vi "Control_Sensing_Sep.vi"() -> ()   [LabVIEW 2019]
uses:
  Control 1.ctl
  <vilib>/myRIO/Instrument Drivers/Onboard IO/I2C/typedefs/I2C User Configuration.ctl
  <vilib>/myRIO/Instrument Drivers/Onboard IO/I2C/typedefs/I2C Transfer Rate.ctl
  <vilib>/myRIO/Instrument Drivers/Onboard IO/I2C/typedefs/I2C Reference.ctl
  <vilib>/myRIO/Common/Instrument Driver Framework/Utilities/typedefs/myRIO Generic Hardware Reference.ctl
  <vilib>/myRIO/Common/Instrument Driver Framework/Utilities/typedefs/Hardware Version Enum.ctl
  <vilib>/myRIO/Common/Instrument Driver Framework/Utilities/typedefs/myRIO v1.0 Reference.ctl
  <vilib>/myRIO/Common/Instrument Driver Framework/Utilities/typedefs/Generic FPGA Reference.ctl
  <vilib>/myRIO/Common/Instrument Driver Framework/myRIO v1.0/I2C/typedefs/I2C Channels Enum.ctl
  <vilib>/myRIO/Instrument Drivers/Onboard IO/I2C/typedefs/I2C Configuration.ctl
  <vilib>/userDefined/High Color/nirio_resource_hc.ctl
  <vilib>/myRIO/Instrument Drivers/Onboard IO/AI/typedefs/AI Reference.ctl
  <vilib>/myRIO/Common/Instrument Driver Framework/myRIO v1.0/AI/typedefs/AI Channels List.ctl
  <vilib>/myRIO/Common/Instrument Driver Framework/myRIO v1.0/AI/typedefs/AI Channels Enum.ctl
  <vilib>/myRIO/Common/Instrument Driver Framework/Utilities/typedefs/Analog Scaling Constants List.ctl
  <vilib>/myRIO/Common/Instrument Driver Framework/Utilities/typedefs/Analog Scaling Constants.ctl
  <vilib>/myRIO/Instrument Drivers/Onboard IO/PWM/typedefs/PWM Reference.ctl
  <vilib>/myRIO/Common/Instrument Driver Framework/myRIO v1.0/PWM/typedefs/PWM Channels Enum.ctl
  <vilib>/myRIO/Instrument Drivers/Onboard IO/PWM/typedefs/PWM Configuration.ctl
  <vilib>/myRIO/Instrument Drivers/Onboard IO/DIO/typedefs/DIO Reference.ctl
  <vilib>/myRIO/Common/Instrument Driver Framework/myRIO v1.0/DIO/typedefs/DIO Channels List.ctl
  <vilib>/myRIO/Common/Instrument Driver Framework/myRIO v1.0/DIO/typedefs/DIO Channels Enum.ctl
  <vilib>/myRIO/Common/Instrument Driver Framework/Utilities/vis/Is FPGA Ref Available.vi
  <vilib>/myRIO/Common/Instrument Driver Framework/myRIO v1.0/I2C/vis/myRIO v1.1 Open I2C.vi
  <vilib>/myRIO/Instrument Drivers/Onboard IO/I2C/vis/Configure.vi
  <vilib>/myRIO/Instrument Drivers/Onboard IO/I2C/vis/Write.vi
  <vilib>/myRIO/Common/Instrument Driver Framework/myRIO v1.0/AI/vis/myRIO v1.1 Open AI.vi
  <vilib>/myRIO/Instrument Drivers/Onboard IO/AI/vis/Read.vi
  <vilib>/myRIO/Common/Instrument Driver Framework/myRIO v1.0/DIO/vis/myRIO v1.1 Open DIO.vi
  <vilib>/myRIO/Instrument Drivers/Onboard IO/DIO/vis/Write.vi
  <vilib>/myRIO/Common/Instrument Driver Framework/myRIO v1.0/PWM/vis/myRIO v1.1 Open PWM.vi
  <vilib>/myRIO/Instrument Drivers/Onboard IO/PWM/vis/Set Duty Cycle and Frequency.vi
  <vilib>/myRIO/Instrument Drivers/Onboard IO/I2C/vis/Write Read.vi
  <vilib>/myRIO/Common/Instrument Driver Framework/myRIO v1.0/UART/vis/myRIO v1.0 Close UART.vi
  <vilib>/myRIO/Common/Instrument Driver Framework/Utilities/vis/Validate Channels.vi
  <vilib>/myRIO/Common/Instrument Driver Framework/myRIO v1.0/I2C/vis/myRIO v1.0 Reserve I2C.vi
  <vilib>/myRIO/Common/Instrument Driver Framework/myRIO v1.0/AI/vis/myRIO v1.0 Reserve AI.vi
  <vilib>/myRIO/Common/Instrument Driver Framework/myRIO v1.0/DIO/vis/myRIO v1.0 Reserve DIO.vi
  <vilib>/myRIO/Common/Instrument Driver Framework/myRIO v1.0/PWM/vis/myRIO v1.0 Reserve PWM.vi
  <vilib>/myRIO/Common/Instrument Driver Framework/myRIO v1.0/I2C/vis/myRIO v1.0 Build MUX Configuration I2C.vi
  <vilib>/myRIO/Common/Instrument Driver Framework/myRIO v1.0/Resource Manager/vis/myRIO v1.0 Reserve Channel List.vi
  <vilib>/myRIO/Common/Instrument Driver Framework/myRIO v1.0/AI/vis/myRIO v1.0 Build MUX Configuration AI.vi
  <vilib>/myRIO/Common/Instrument Driver Framework/myRIO v1.0/DIO/vis/myRIO v1.0 Build MUX Configuration DIO.vi
  <vilib>/myRIO/Common/Instrument Driver Framework/myRIO v1.0/PWM/vis/myRIO v1.0 Build MUX Configuration PWM.vi
  <vilib>/myRIO/Common/Instrument Driver Framework/myRIO v1.0/Resource Manager/vis/myRIO v1.0 Create Configuration List.vi
  <vilib>/myRIO/Common/Instrument Driver Framework/myRIO v1.0/Resource Manager/vis/myRIO v1.0 Reserve Channel.vi
  <vilib>/myRIO/Common/Instrument Driver Framework/myRIO v1.0/Resource Manager/vis/myRIO v1.0 Unreserve Channel.vi
  <vilib>/myRIO/Common/Instrument Driver Framework/myRIO v1.0/Resource Manager/vis/myRIO v1.0 Build Mutex Name.vi
  <vilib>/imath/engines/lvmath2/RunTimeEngine/NodeEndStatement/NIMS_NodeEndStatement_Output.vi
  <instcachedir>/0/NIMS_NodeEndStatement_Output_53EC0D466D134D7ABD903AC30B43404B.lvgen/NIMS_NodeEndStatement_Output_53EC0D466D134D7ABD903AC30B43404B_000.vi
  <instcachedir>/0/NIMS_NodeEndStatement_Output_53EC0D466D134D7ABD903AC30B43404B.lvgen/NIMS_NodeEndStatement_Output_53EC0D466D134D7ABD903AC30B43404B_005.vi
  <vilib>/imath/engines/lvmath2/RunTimeEngine/ErrorHandling/NIMS_Finalize Error.vi
  <vilib>/imath/engines/lvmath2/RunTimeEngine/BuiltInFunctions/length/NIMS_length(GV).vi
  <instcachedir>/0/NIMS_length(GV)_08A3D13377FD4E4B96F5795FBF3698FA.lvgen/NIMS_length(GV)_08A3D13377FD4E4B96F5795FBF3698FA_000.vi
  <vilib>/imath/engines/lvmath2/RunTimeEngine/BuiltInFunctions/ones/NIMS_V=ones(I32,I32).vi
  <vilib>/imathl/engines/lvmath/Functions/Error Handling/Create Error.vi
  <vilib>/imath/engines/lvmath2/RunTimeEngine/RangeToken/NIMS_Range.vi
  <instcachedir>/0/NIMS_Range_FADF6ADDA3E145BB934C8BD4C7DAAB97.lvgen/NIMS_Range_FADF6ADDA3E145BB934C8BD4C7DAAB97_000.vi
  <vilib>/imath/engines/lvmath2/RunTimeEngine/Managers/WorkSpace/UID Generator.vi
  <vilib>/imath/engines/lvmath2/RunTimeEngine/RunTimeType/NIMS_RunTimeType_From StrictType (excl LVString).vi
  <instcachedir>/0/NIMS_RunTimeType_From StrictType (excl LVString)_D8AFBA86A94845AAA577C895450664BD.lvgen/NIMS_RunTimeType_From StrictType (excl LVString)_D8AFBA86A94845AAA577C895450664BD_000.vi
  <vilib>/imath/engines/lvmath2/RunTimeEngine/LocalVariableDefStatement/MC_LocalVariableDefStatement_Display.vi
  <vilib>/imath/engines/lvmath2/RunTimeEngine/BuiltInFunctions/diag/NIMS_diag.vi
  <instcachedir>/0/NIMS_diag_DCAB8C8FDAF64F9E84492BB524435AA9.lvgen/NIMS_diag_DCAB8C8FDAF64F9E84492BB524435AA9_003.vi
  <vilib>/imath/engines/lvmath2/RunTimeEngine/BuiltInFunctions/mirrorh/NIMS_mirrorh(GM).vi
  <instcachedir>/0/NIMS_mirrorh(GM)_A650AD0D730A4A8EBE251B4C5C7CA115.lvgen/NIMS_mirrorh(GM)_A650AD0D730A4A8EBE251B4C5C7CA115_004.vi
  <vilib>/imath/engines/lvmath2/RunTimeEngine/RowToken/NIMS_RowToken_M_M.vi
  <instcachedir>/0/NIMS_RowToken_M_M_21FE36D058524603B8B587AC30FD72C2.lvgen/NIMS_RowToken_M_M_21FE36D058524603B8B587AC30FD72C2_005.vi
  <vilib>/imath/engines/lvmath2/RunTimeEngine/ErrorHandling/NIMS_Create Error From Enums.vi
  <vilib>/imath/engines/lvmath2/RunTimeEngine/Managers/SymbolTable/Clear UID.vi
  <instcachedir>/0/NIMS_NodeEndStatement_Output_53EC0D466D134D7ABD903AC30B43404B.lvgen/NIMS_NodeEndStatement_Output_53EC0D466D134D7ABD903AC30B43404B_002.vi
  <instcachedir>/0/NIMS_NodeEndStatement_Output_53EC0D466D134D7ABD903AC30B43404B.lvgen/NIMS_NodeEndStatement_Output_53EC0D466D134D7ABD903AC30B43404B_010.vi
  <vilib>/Utility/VariantDataType/GetNumericInfo.vi
  <vilib>/Utility/error.llb/Error Cluster From Error Code.vi
  <vilib>/myRIO/Common/Instrument Driver Framework/myRIO v1.0/myRIO v1.1 Open.vi
  <vilib>/myRIO/Common/Instrument Driver Framework/Utilities/vis/IO Manager.vi
  <vilib>/myRIO/Common/Instrument Driver Framework/Utilities/vis/Configuration Manager.vi
  <vilib>/myRIO/Common/Instrument Driver Framework/myRIO v1.0/Resource Manager/vis/myRIO v1.0 Configure IO.vi
  <vilib>/myRIO/Common/Instrument Driver Framework/myRIO v1.0/myRIO v1.0 Close.vi
  <vilib>/myRIO/Common/Instrument Driver Framework/myRIO v1.0/I2C/vis/myRIO v1.0 Configure I2C.vi
  <vilib>/myRIO/Common/Instrument Driver Framework/myRIO v1.0/I2C/vis/myRIO v1.0 Write I2C.vi
  <vilib>/myRIO/Common/Instrument Driver Framework/myRIO v1.0/AI/vis/myRIO v1.0 Get Scaling Constants AI.vi
  <vilib>/myRIO/Common/Instrument Driver Framework/myRIO v1.0/AI/vis/myRIO v1.0 Read AI.vi
  <vilib>/myRIO/Common/Instrument Driver Framework/myRIO v1.0/PWM/vis/myRIO v1.0 Write PWM.vi
  <vilib>/myRIO/Common/Instrument Driver Framework/myRIO v1.0/DIO/vis/myRIO v1.0 Write DIO.vi
  <vilib>/myRIO/Common/Instrument Driver Framework/myRIO v1.0/I2C/vis/myRIO v1.0 Read I2C.vi
  OneDrive/Documents/LabVIEW Data/MathScriptVIs/MCStatic_41946317732_39d282e6f644b4de5e03d5ec5e14f762.vi
  <instcachedir>/0/MCStatic_41946317732_39d282e6f644b4de5e03d5ec5e14f762_F82D6288F92F4DD7BE24A1113A5A915E.lvgen/MCStatic_41946317732_39d282e6f644b4de5e03d5ec5e14f762_F82D6288F92F4DD7BE24A1113A5A915E_000.vi
  <vilib>/imath/engines/lvmath2/RunTimeEngine/ArithmeticOperatorToken/NIMS_ArithmeticOperator_multmx.vi
  <instcachedir>/0/NIMS_ArithmeticOperator_multmx_77F1D2D6F4D94BA7A97C4E7185C02392.lvgen/NIMS_ArithmeticOperator_multmx_77F1D2D6F4D94BA7A97C4E7185C02392_003.vi
  <instcachedir>/0/NIMS_diag_DCAB8C8FDAF64F9E84492BB524435AA9.lvgen/NIMS_diag_DCAB8C8FDAF64F9E84492BB524435AA9_002.vi
  <vilib>/imath/engines/lvmath2/RunTimeEngine/BuiltInFunctions/max/1 input/NIMS_max(CM).vi
  <instcachedir>/0/NIMS_max(CM)_ECFF9CEF2CF74B92B05BC258ECD38873.lvgen/NIMS_max(CM)_ECFF9CEF2CF74B92B05BC258ECD38873_000.vi
  <vilib>/imath/engines/lvmath/Functions/Error Handling/MergeErrorsWrapper.vi
  <vilib>/imath/engines/lvmath2/RunTimeEngine/CommandStatement/MC_CommandStatement_break.vi
  OneDrive/Documents/LabVIEW Data/MathScriptVIs/MCStatic_41946317732_3e71c9587ee176df8890ce07400746a8.vi
  <instcachedir>/0/MCStatic_41946317732_3e71c9587ee176df8890ce07400746a8_07A171384687481495CD1245C64FEFFE.lvgen/MCStatic_41946317732_3e71c9587ee176df8890ce07400746a8_07A171384687481495CD1245C64FEFFE_002.vi
  <vilib>/imath/engines/lvmath2/RunTimeEngine/ArithmeticOperatorToken/NIMS_ArithmeticOperator_minus.vi
  <instcachedir>/0/NIMS_ArithmeticOperator_minus_12BFF9710EA5430A9EE87C5BC3F65186.lvgen/NIMS_ArithmeticOperator_minus_12BFF9710EA5430A9EE87C5BC3F65186_009.vi
  <vilib>/imath/engines/lvmath2/RunTimeEngine/BuiltInFunctions/norm/NIMS_norm(GM,DBL).vi
  <instcachedir>/0/NIMS_norm(GM,DBL)_8BCB088F207E48DF95CF5C1DC502F84D.lvgen/NIMS_norm(GM,DBL)_8BCB088F207E48DF95CF5C1DC502F84D_001.vi
  <vilib>/imath/engines/lvmath2/RunTimeEngine/BuiltInFunctions/abs/NIMS_abs(signed).vi
  <instcachedir>/0/NIMS_abs(signed)_C4FCB8E6058B49B797C7C8D53CA5F6EC.lvgen/NIMS_abs(signed)_C4FCB8E6058B49B797C7C8D53CA5F6EC_003.vi
  <vilib>/imath/engines/lvmath2/RunTimeEngine/BuiltInFunctions/max/1 input/NIMS_max(RM).vi
  <instcachedir>/0/NIMS_max(RM)_0B4294876EE440609D638D7C5C6E788E.lvgen/NIMS_max(RM)_0B4294876EE440609D638D7C5C6E788E_000.vi
  <vilib>/imath/engines/lvmath2/RunTimeSupport/NIMS_Get Scalar_w Error.vi
  <instcachedir>/0/NIMS_Get Scalar_w Error_90FA09EFB1C84794B43793796939E0E3.lvgen/NIMS_Get Scalar_w Error_90FA09EFB1C84794B43793796939E0E3_010.vi
  <vilib>/imath/engines/lvmath2/RunTimeEngine/BuiltInFunctions/eye/NIMS_M=eye(I32).vi
  <instcachedir>/0/NIMS_ArithmeticOperator_multmx_77F1D2D6F4D94BA7A97C4E7185C02392.lvgen/NIMS_ArithmeticOperator_multmx_77F1D2D6F4D94BA7A97C4E7185C02392_007.vi
  <vilib>/imath/engines/lvmath2/RunTimeEngine/ArithmeticOperatorToken/NIMS_ArithmeticOperator_plus.vi
  <instcachedir>/0/NIMS_ArithmeticOperator_plus_5C9385B0197D46E2B844C41E02F9EC39.lvgen/NIMS_ArithmeticOperator_plus_5C9385B0197D46E2B844C41E02F9EC39_002.vi
  <vilib>/imath/engines/lvmath2/RunTimeEngine/ArithmeticOperatorToken/NIMS_ArithmeticOperator_leftdivmx(C,C).vi
  <instcachedir>/0/NIMS_ArithmeticOperator_leftdivmx(C,C)_FFA86DC98B994D28AA7593516F1DAFDA.lvgen/NIMS_ArithmeticOperator_leftdivmx(C,C)_FFA86DC98B994D28AA7593516F1DAFDA_000.vi
  <vilib>/imath/engines/lvmath2/RunTimeEngine/ArithmeticOperatorToken/NIMS_ArithmeticOperator_rightdiv.vi
  <instcachedir>/0/NIMS_ArithmeticOperator_rightdiv_23AAA10E4B1E4564B1AF1956090A34B0.lvgen/NIMS_ArithmeticOperator_rightdiv_23AAA10E4B1E4564B1AF1956090A34B0_004.vi
  <instcachedir>/0/NIMS_ArithmeticOperator_minus_12BFF9710EA5430A9EE87C5BC3F65186.lvgen/NIMS_ArithmeticOperator_minus_12BFF9710EA5430A9EE87C5BC3F65186_008.vi
  <vilib>/imath/engines/lvmath2/RunTimeEngine/ArithmeticOperatorToken/NIMS_ArithmeticOperator_rightdivmx(C,C).vi
  <instcachedir>/0/NIMS_ArithmeticOperator_rightdivmx(C,C)_4C9834AF73264B85B2EC0ABB36B07CCF.lvgen/NIMS_ArithmeticOperator_rightdivmx(C,C)_4C9834AF73264B85B2EC0ABB36B07CCF_000.vi
  <vilib>/imath/engines/lvmath2/RunTimeEngine/ArithmeticOperatorToken/NIMS_ArithmeticOperator_powermx(M,M).vi
  <vilib>/imath/engines/lvmath2/RunTimeEngine/BuiltInFunctions/max/2 inputs/NIMS_max(CG,CG)-no size check.vi
  <instcachedir>/0/NIMS_max(CG,CG)-no size check_0D8807EB624448B1961BA94FD6C7666D.lvgen/NIMS_max(CG,CG)-no size check_0D8807EB624448B1961BA94FD6C7666D_000.vi
  <instcachedir>/0/MCStatic_41946317732_39d282e6f644b4de5e03d5ec5e14f762_F82D6288F92F4DD7BE24A1113A5A915E.lvgen/MCStatic_41946317732_39d282e6f644b4de5e03d5ec5e14f762_F82D6288F92F4DD7BE24A1113A5A915E_002.vi
  <vilib>/imath/engines/lvmath2/RunTimeEngine/CommandStatement/NIMS_CommandStatement_MaskErr.vi
  <vilib>/imath/engines/lvmath2/RunTimeEngine/NodeEndStatement/NIMS_NodeEndStatement_Get Vector.vi
  <instcachedir>/0/NIMS_NodeEndStatement_Get Vector_92F29E6578CC4FEABDAC0B727A70E862.lvgen/NIMS_NodeEndStatement_Get Vector_92F29E6578CC4FEABDAC0B727A70E862_003.vi
  OneDrive/Documents/LabVIEW Data/MathScriptVIs/MCStatic_41946317732_98df4686c37d1a1eae0c5985e9f7cbe2.vi
  <instcachedir>/0/MCStatic_41946317732_98df4686c37d1a1eae0c5985e9f7cbe2_A0FFC33B284B421AAD6E5346CB265B3A.lvgen/MCStatic_41946317732_98df4686c37d1a1eae0c5985e9f7cbe2_A0FFC33B284B421AAD6E5346CB265B3A_001.vi
  OneDrive/Documents/LabVIEW Data/MathScriptVIs/MCStatic_41946317732_460fc674ac509ba7029ac98c4ab25738.vi
  <instcachedir>/0/MCStatic_41946317732_460fc674ac509ba7029ac98c4ab25738_40677AF033AE4176B404E9AC0BBDDC84.lvgen/MCStatic_41946317732_460fc674ac509ba7029ac98c4ab25738_40677AF033AE4176B404E9AC0BBDDC84_001.vi
  <instcachedir>/0/MCStatic_41946317732_98df4686c37d1a1eae0c5985e9f7cbe2_A0FFC33B284B421AAD6E5346CB265B3A.lvgen/MCStatic_41946317732_98df4686c37d1a1eae0c5985e9f7cbe2_A0FFC33B284B421AAD6E5346CB265B3A_003.vi
  <vilib>/myRIO/Common/Instrument Driver Framework/Utilities/vis/FPGA Ref Manager.vi
  <vilib>/myRIO/Common/Instrument Driver Framework/myRIO v1.0/myRIO v1.0 Reset FPGA.vi
  <vilib>/myRIO/Common/Instrument Driver Framework/myRIO v1.0/IRQ/vis/myRIO v1.0 IRQ Info FGV.vi
  <vilib>/myRIO/Common/Instrument Driver Framework/myRIO v1.0/IRQ/vis/myRIO v1.0 Timer IRQ Info FGV.vi
  <vilib>/myRIO/Common/Instrument Driver Framework/myRIO v1.0/IRQ/vis/myRIO v1.0 ISR Agent.vi
  <vilib>/myRIO/Instrument Drivers/Utilities/vis/Reset Index.vi
  <vilib>/myRIO/Common/Instrument Driver Framework/myRIO v1.0/Resource Manager/vis/myRIO v1.0 Block Write Resource Manager.vi
  <vilib>/myRIO/Express VI/Onboard IO/I2C/I2C Express VI.xnode
  <vilib>/myRIO/Instrument Drivers/Onboard IO/I2C/vis/myRIO I2C Open.xnode
  <vilib>/myRIO/Express VI/Onboard IO/AI/AI Express VI.xnode
  <vilib>/myRIO/Instrument Drivers/Onboard IO/AI/vis/myRIO AI Open.xnode
  <vilib>/myRIO/Express VI/Onboard IO/PWM/PWM Express VI.xnode
  <vilib>/myRIO/Instrument Drivers/Onboard IO/PWM/vis/myRIO PWM Open.xnode
  <vilib>/myRIO/Express VI/Onboard IO/DO/DO Express VI.xnode
  <vilib>/myRIO/Instrument Drivers/Onboard IO/DIO/vis/myRIO DIO Open.xnode
  magnetic_sensing-main/Analytic_Jacobian_Mag_cir_array_noM.m
  magnetic_sensing-main/PM_forward_field_noM.m
  magnetic_sensing-main/Analytic_Jacobian_Mag_cir_array_test.m
  magnetic_sensing-main/PM_forward_field.m
  <vilib>/myRIO/Instrument Drivers/Onboard IO/I2C/I2C.lvlib
  <vilib>/myRIO/Instrument Drivers/Utilities/Utilities.lvlib
  <instcachedir>/0/MCStatic_41946317732_460fc674ac509ba7029ac98c4ab25738_40677AF033AE4176B404E9AC0BBDDC84.lvgen/MCStatic_41946317732_460fc674ac509ba7029ac98c4ab25738_40677AF033AE4176B404E9AC0BBDDC84_003.vi
  <vilib>/myRIO/Instrument Drivers/Onboard IO/PWM/PWM.lvlib
  <vilib>/myRIO/Instrument Drivers/Onboard IO/DIO/DIO.lvlib
  <instcachedir>/0/MCStatic_41946317732_3e71c9587ee176df8890ce07400746a8_07A171384687481495CD1245C64FEFFE.lvgen/MCStatic_41946317732_3e71c9587ee176df8890ce07400746a8_07A171384687481495CD1245C64FEFFE_000.vi
  <vilib>/imath/engines/lvmath2/RunTimeEngine/Managers/SymbolTable/NIMS_WorkSpace.lvlib
  <vilib>/myRIO/Instrument Drivers/Onboard IO/AI/AI.lvlib
panel:
  out "Encoder 2 AI1":dbl
  out "Encoder 1 AI0":dbl
  out "Sensing time":u32
  in  "Bifur?":bool
  in  "M":dbl
  in  "Update M in realtime?":bool
  in  "Clear plot?":bool
  out "pm_hat_opt":dbl[](array[numeric])
  in  "stop":bool
  in  "Actuation Current":dbl(slide) scale=-1.0..1.0
  in  "Actuation on?":bool
  in  "Action Mode":T1=enum."Sensing"
  out "XY Graph":cluster{dbl[], dbl[]}[](graph)
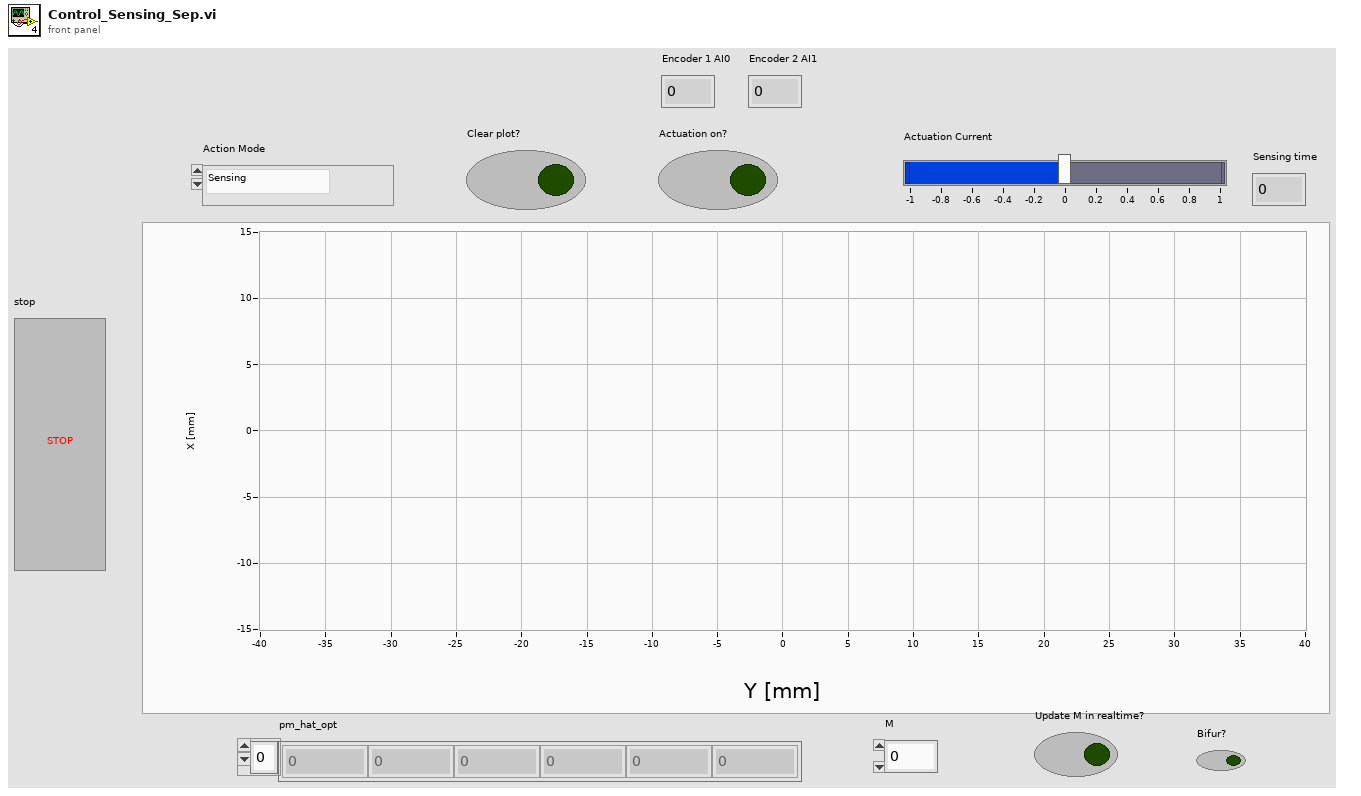
[diagram p1: front panel]
types:
  T1 = typedef "Control 1.ctl" = enum16{"Actuation", "Waiting", "Sensing"}
  T2 = typedef "I2C.lvlib/I2C Reference.ctl" = cluster{"myRIO Reference":T3, "I2C Channels Enum":T7, "I2C Configuration":T8}
  T3 = typedef "myRIO Generic Hardware Reference.ctl" = cluster{"myRIO Model":T4, "myRIO Hardware Reference":T5}
  T4 = typedef "Hardware Version Enum.ctl" = enum16{"Unknown", "myRIO-1900", "myRIO-1950", "roboRIO", "NI ELVIS RIO CM", "ELVIS III"}
  T5 = typedef "myRIO v1.0 Reference.ctl" = cluster{"Generic FPGA Reference":T6, "Allow multiple opens":bool}
  T6 = typedef "Generic FPGA Reference.ctl" = refnum<k20>
  T7 = typedef "I2C Channels Enum.ctl" = enum16{"Not Connected", "A/I2C", "B/I2C", "I2C/I2C"}
  T8 = typedef "I2C.lvlib/I2C Configuration.ctl" = cluster{"I2C Transfer Rate":T9}
  T9 = typedef "I2C.lvlib/I2C Transfer Rate.ctl" = enum16{"Standard mode (100 kbps)", "Fast mode (400 kbps)"}
  T10 = typedef "I2C.lvlib/I2C User Configuration.ctl" = cluster{"I2C Transfer Rate":T9}
  T11 = typedef "nirio_resource_hc.ctl" = tag
  T12 = typedef "DIO.lvlib/DIO Reference.ctl" = cluster{"myRIO Reference":T3, "DIO Channels List":T13}
  T13 = typedef "DIO Channels List.ctl" = T14[]
  T14 = typedef "DIO Channels Enum.ctl" = enum16{"Not Connected", "C/DIO0", "C/DIO1", "C/DIO2", "C/DIO3", "C/DIO4", "C/DIO5", "C/DIO6", "C/DIO7", "A/DIO0", "A/DIO1", "A/DIO2", "A/DIO3", "A/DIO4", "A/DIO5", "A/DIO6", "A/DIO7", "A/DIO8", "A/DIO9", "A/DIO10", "A/DIO11", "A/DIO12", "A/DIO13", "A/DIO14", "A/DIO15", "A/DIO16", "A/DIO17", "A/DIO18", "A/DIO19", "B/DIO0", "B/DIO1", "B/DIO2", "B/DIO3", "B/DIO4", "B/DIO5", "B/DIO6", "B/DIO7", "B/DIO8", "B/DIO9", "B/DIO10", "B/DIO11", "B/DIO12", "B/DIO13", "B/DIO14", "B/DIO15", "B/DIO16", "B/DIO17", "B/DIO18", "B/DIO19", "LED0", "LED1", "LED2", "LED3", "Button0", "DIO/DIO0", "DIO/DIO1", "DIO/DIO2", "DIO/DIO3", "DIO/DIO4", "DIO/DIO5", "DIO/DIO6", "DIO/DIO7", "DIO/DIO8", "DIO/DIO9", "SPI/CS0", "SPI/CS1", "SPI/CS2", "SPI/CS3", "LED RADIO (Green)", "LED RADIO (Red)", "LED COMM (Green)", "LED COMM (Red)", "LED MODE (Green)", "LED MODE (Red)"}
  T15 = typedef "PWM.lvlib/PWM Reference.ctl" = cluster{"myRIO Reference":T3, "PWM Channels Enum":T16, "PWM Configuration":T17}
  T16 = typedef "PWM Channels Enum.ctl" = enum16{"Not Connected", "C/PWM0", "C/PWM1", "A/PWM0", "A/PWM1", "A/PWM2", "A/PWM3", "A/PWM4", "A/PWM5", "A/PWM6", "A/PWM7", "A/PWM8", "A/PWM9", "A/PWM10", "A/PWM11", "A/PWM12", "A/PWM13", "A/PWM14", "A/PWM15", "A/PWM16", "A/PWM17", "A/PWM18", "A/PWM19", "B/PWM0", "B/PWM1", "B/PWM2", "B/PWM3", "B/PWM4", "B/PWM5", "B/PWM6", "B/PWM7", "B/PWM8", "B/PWM9", "B/PWM10", "B/PWM11", "B/PWM12", "B/PWM13", "B/PWM14", "B/PWM15", "B/PWM16", "B/PWM17", "B/PWM18", "B/PWM19", "PWM/PWM0", "PWM/PWM1", "PWM/PWM2", "PWM/PWM3", "PWM/PWM4", "PWM/PWM5", "PWM/PWM6", "PWM/PWM7", "PWM/PWM8", "PWM/PWM9"}
  T17 = typedef "PWM.lvlib/PWM Configuration.ctl" = cluster{"Frequency":dbl, "Duty Cycle":dbl}
  T18 = typedef "AI.lvlib/AI Reference.ctl" = cluster{"myRIO Reference":T3, "AI Channels List":T19, "AI Scaling Constants List":T21}
  T19 = typedef "AI Channels List.ctl" = T20[]
  T20 = typedef "AI Channels Enum.ctl" = enum16{"Not Connected", "AudioIn/Left", "AudioIn/Right", "C/AI0", "C/AI1", "A/AI0", "A/AI1", "A/AI2", "A/AI3", "A/AI4", "A/AI5", "A/AI6", "A/AI7", "B/AI0", "B/AI1", "B/AI2", "B/AI3", "B/AI4", "B/AI5", "B/AI6", "B/AI7", "AI/AI0", "AI/AI1", "AI/AI2", "AI/AI3", "A/AI0 (DIFF)", "A/AI1 (DIFF)", "A/AI2 (DIFF)", "A/AI3 (DIFF)", "B/AI0 (DIFF)", "B/AI1 (DIFF)", "B/AI2 (DIFF)", "B/AI3 (DIFF)"}
  T21 = typedef "Analog Scaling Constants List.ctl" = T22[]
  T22 = typedef "Analog Scaling Constants.ctl" = cluster{"LSB Weight (Volts)":dbl, "Offset (Volts)":dbl, "Signed?":bool}
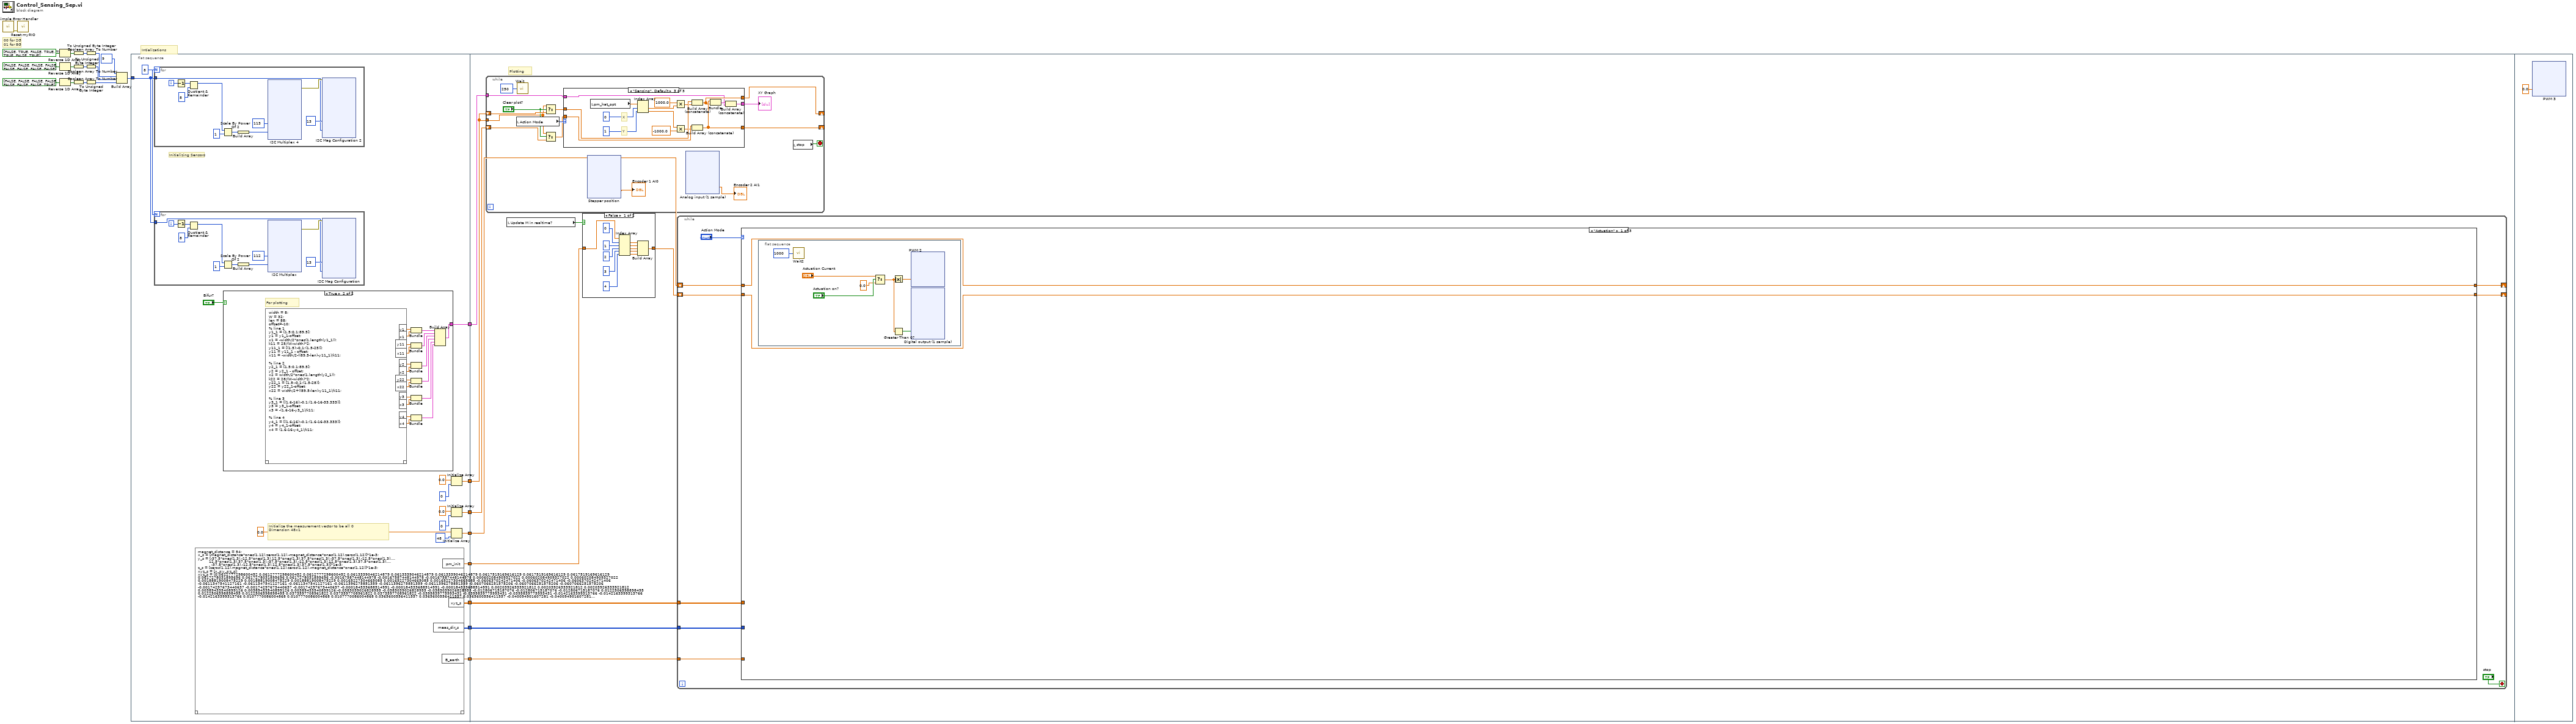
[diagram p0: block diagram]
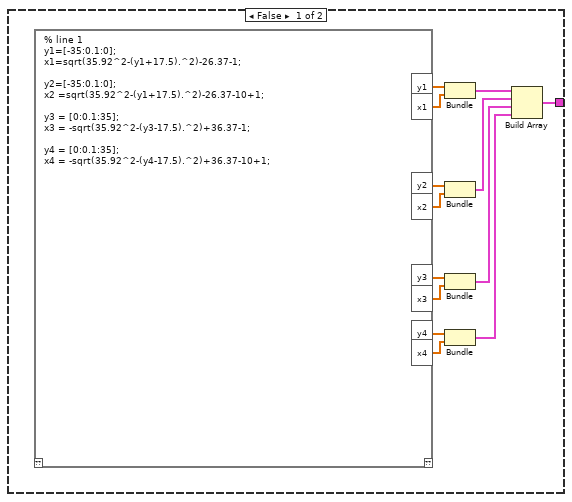
[diagram p2: hidden frame]
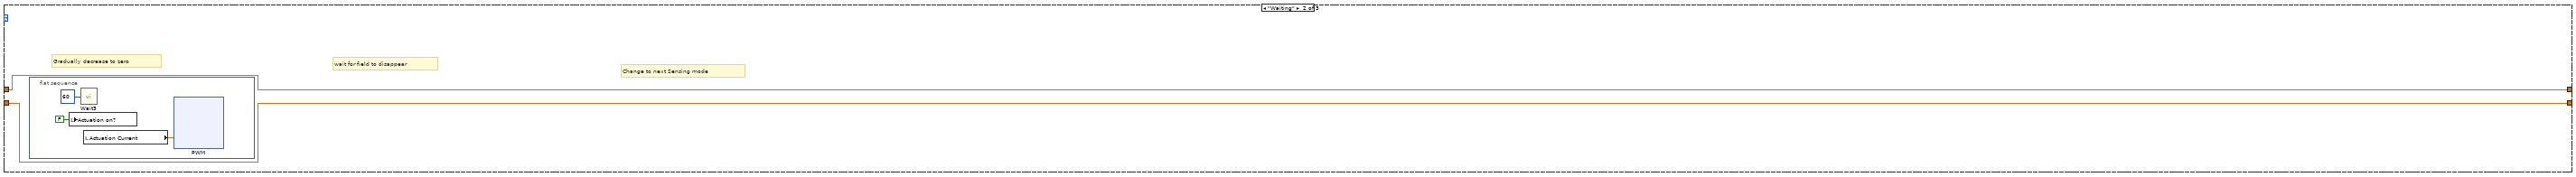
[diagram p4: hidden frame]
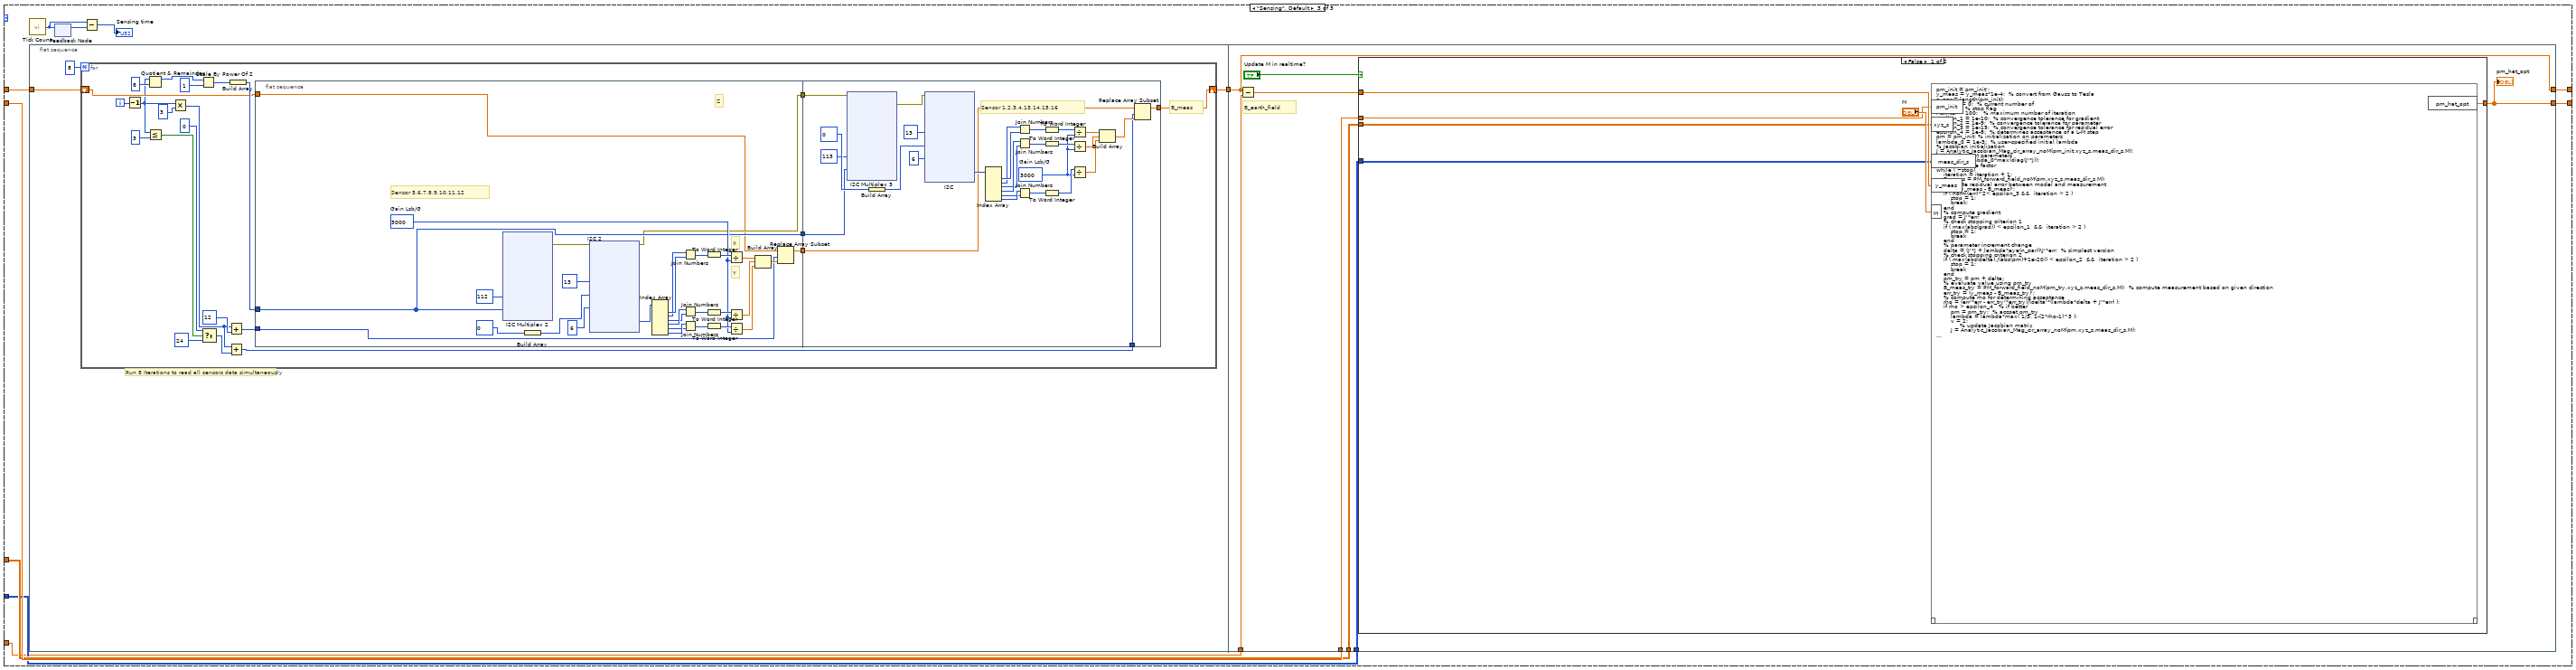
[diagram p5: hidden frame]
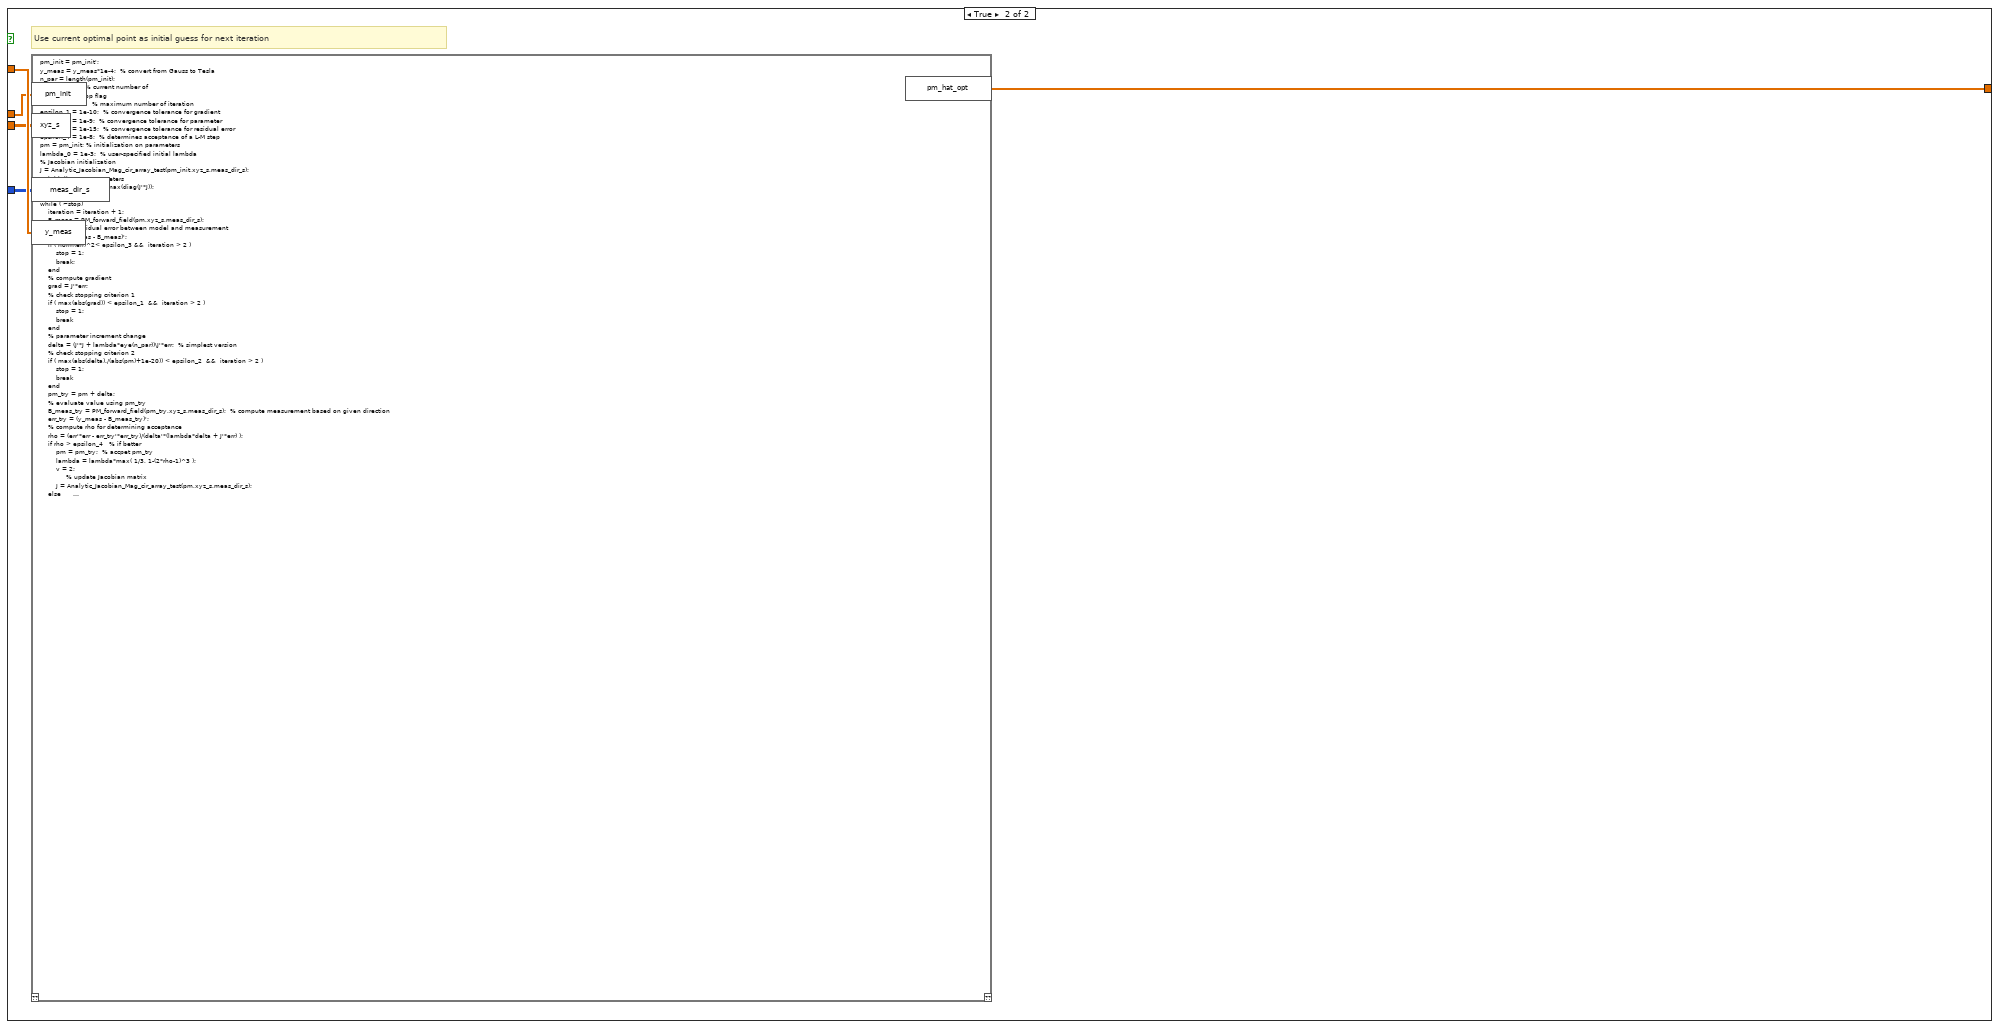
[diagram p6: hidden frame]
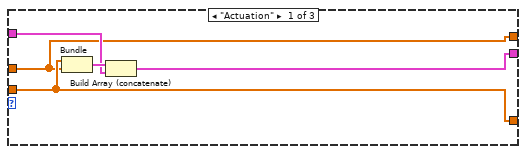
[diagram p7: hidden frame]
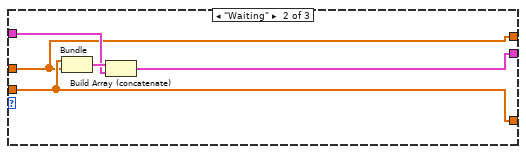
[diagram p8: hidden frame]
diagram:
  # "Intializations"
  # "00 for 2G\n01 for 8G"
  n1 = call <vilib>:"Simple Error Handler.vi"() -> ("error out"=w4:errorcluster)  [unwired: 5 in, 4 out]
  n2 = call <vilib>:"Reset myRIO.vi"("error in (no error)"=w4) -> ()  [unwired: 10 in, 1 out]
  n3 = Reverse 1D Array(array=bool[] [FALSE, TRUE, FALSE, TRUE, TRUE, TRUE, FALSE, TRUE]) -> (reversed array=w17:bool[])
  n4 = Reverse 1D Array(array=bool[] [FALSE, FALSE, FALSE, FALSE, FALSE, FALSE, FALSE, FALSE]) -> (reversed array=w16:bool[])
  n5 = Reverse 1D Array(array=bool[] [FALSE, FALSE, FALSE, FALSE, FALSE, FALSE, FALSE, TRUE]) -> (reversed array=w14:bool[])
  n6 = Boolean Array To Number(Boolean array=w17) -> (number=w11:u32)
  n7 = Boolean Array To Number(Boolean array=w16) -> (number=w10:u32)
  n8 = Boolean Array To Number(Boolean array=w14) -> (number=w9:u32)
  n9 = To Unsigned Byte Integer(number=w11) -> (unsigned 8bit integer=w8:u8)
  n10 = To Unsigned Byte Integer(number=w10) -> (unsigned 8bit integer=w7:u8)
  n11 = To Unsigned Byte Integer(number=w9) -> (unsigned 8bit integer=w6:u8)
  n12 = Build Array(u8 9 ("address"), w8, w7, w6) -> (w5:u8[])
  n13 = flat-sequence {
    tunnel: w5 -> [w40]
    tunnel: [w38] -> w23
    tunnel: [w37] -> w22
    tunnel: [w34] -> w21
    tunnel: [w33] -> w20
    tunnel: [w32] -> w19
    tunnel: [w27] -> w3
    tunnel: [w26] -> w2
    tunnel: [w25] -> w1
    tunnel: w23 -> [w995]
    tunnel: w22 -> [w996]
    tunnel: w21 -> [w997]
    tunnel: w20 -> [w990]
    tunnel: w19 -> [w994]
    tunnel: w3 -> [w993]
    tunnel: w2 -> [w991]
    tunnel: w1 -> [w992]
    frame #0 {
      w39 = 8
      # "Initialize the measurement vector to be all 0\nDimension 48x1"
      # "Initializing Sensors"
      n14 = for {
        N: w39 -> [_]
        tunnel: w40 -> [w821]
        i -> [w815]
        n15 = Decrement(x=w815) -> (x-1=w814:i32)
        n16 = Quotient & Remainder(x=w814, y=8) -> (x-y*floor(x/y)=w816:i32)  [unwired: 1 out]
        n17 = Scale By Power Of 2(n=w816, x=1) -> (x*2^n=w818:i32)
        n18 = Build Array(w818) -> (w824:i32[])
        n19 = xnode "I2C Multiplex 4"("Slave Address (7-bit)"=u8 113, "Bytes to Write"=w824) -> ("error out"=w823:errorcluster)  [unwired: 1 in]
        n20 = xnode "I2C Mag Configuration 2"("Slave Address (7-bit)"=u8 13, "Bytes to Write"=w821, "error in (no error)"=w823) -> ()  [unwired: 1 out]
      }
      n21 = for {
        N: w39 -> [_]
        tunnel: w40 -> [w908]
        i -> [w902]
        n22 = Decrement(x=w902) -> (x-1=w901:i32)
        n23 = Quotient & Remainder(x=w901, y=8) -> (x-y*floor(x/y)=w903:i32)  [unwired: 1 out]
        n24 = Scale By Power Of 2(n=w903, x=1) -> (x*2^n=w905:i32)
        n25 = Build Array(w905) -> (w911:i32[])
        n26 = xnode "I2C Multiplex"("Slave Address (7-bit)"=u8 112, "Bytes to Write"=w911) -> ("error out"=w910:errorcluster)  [unwired: 1 in]
        n27 = xnode "I2C Mag Configuration"("Slave Address (7-bit)"=u8 13, "Bytes to Write"=w908, "error in (no error)"=w910) -> ()  [unwired: 1 out]
      }
      n28 = mathscript code="magnet_distance = 54;\nx_s = [magnet_distance*ones(1,12),zeros(1,12),-magnet_distance*ones(1,12),zeros(1,12)]*1e-3; \ny_s = [-37.5*ones(1,3),-12.5*ones(1,3),12.5*ones(1,3),37.5*ones(1,3),-37.5*ones(1,3),-12.5*ones(1,3),...\n         12.5*ones(1,3),37.5*ones(1,3),-37.5*ones(1,3),-12.5*ones(1,3),12.5*ones(1,3),37.5*ones(1,3),...\n           -37.5*ones(1,3),-12.5*ones(1,3),12.5*ones(1,3),37.5*ones(1,3)]*1e-3; \nz_s = [zeros(1,12),magnet_distance*ones(1,12),zeros(1,12),-magnet_distance*ones(1,12)]*1e-3; \nxyz_s = [x_s;y_s;z_s];  \nxyz_s = [0.0612777298600452 0.0612777298600452 0.0612777298600452 0.0613339046214879 0.0613339046214879 0.0613339046214879 0.0617519169616129 0.0617519169616129 0.0617519169616129 0.0617278031895696 0.0617278031895696 0.0617278031895696 -0.00167587448144978 -0.00167587448144978 -0.00167587448144978 0.000602084909327022 0.000602084909327022 0.000602084909327022 0.00188819008475229 0.00188819008475229 0.00188819008475229 0.00165227304665085 0.00165227304665085 0.00165227304665085 -0.0606370242471406 -0.0606370242471406 -0.0606370242471406 -0.0611347541127161 -0.0611347541127161 -0.0611347541127161 -0.0611396275851359 -0.0611396275851359 -0.0611396275851359 -0.0607066251575206 -0.0607066251575206 -0.0607066251575206 -0.00174297673440637 -0.00174297673440637 -0.00174297673440637 -0.000184533688514991 -0.000184533688514991 -0.000184533688514991 0.00203926333921812 0.00203926333921812 0.00203926333921812 0.00389433540899126 0.00389433540899126 0.00389433540899126;-0.0383039026828955 -0.0383039026828955 -0.0383039026828955 -0.012806715187076 -0.012806715187076 -0.012806715187076 0.0122506598898495 0.0122506598898495 0.0122506598898495 0.0373597708961822 0.0373597708961822 0.0373597708961822 -0.0395839775993431 -0.0395839775993431 -0.0395839775993431 -0.0142163399313766 -0.0142163399313766 -0.0142163399313766 0.0107770086004868 0.0107770086004868 0.0107770086004868 0.0365600556411557 0.0365600556411557 0.0365600556411557 -0.040094901607281 -0.040094901607281 -0.040094901607281 -0.0149090266343068 -0.0149090266343068 -0.0149090266343068 0.0107078118967093 0.0107078118967093 0.0107078118967093 0.0356978973873521 0.0356978973873521 0.0356978973873521 -0.0392056799428433 -0.0392056799428433 -0.0392056799428433 -0.0139322320487061 -0.0139322320487061 -0.0139322320487061 0.0112429513248133 0.0112429513248133 0.0112429513248133 0.0361205812401305 0.0361205812401305 0.0361205812401305;0.00307213814961651 0.00307213814961651 0.00307213814961651 0.0033242461093476 0.0033242461093476 0.0033242461093476 0.00389293419390068 0.00389293419390068 0.00389293419390068 0.00390199978115286 0.00390199978115286 0.00390199978115286 0.0640688323293379 0.0640688323293379 0.0640688323293379 0.0636929900573754 0.0636929900573754 0.0636929900573754 0.0635181326061399 0.0635181326061399 0.0635181326061399 0.0633759954094267 0.0633759954094267 0.0633759954094267 -0.00381527257187291 -0.00381527257187291 -0.00381527257187291 -0.00312975643341264 -0.00312975643341264 -0.00312975643341264 -0.00272771938684928 -0.00272771938684928 -0.00272771938684928 -0.00268843620404175 -0.00268843620404175 -0.00268843620404175 -0.0628805002941716 -0.0628805002941716 -0.0628805002941716 -0.063138590462401 -0.063138590462401 -0.063138590462401 -0.063695098330538 -0.063695098330538 -0.063695098330538 -0.0638823957044235 -0.0638823957044235 -0.0638823957044235]\nmeas_dir_s = [mirrorh(diag([1;-1;1])),...\n              mirrorh(diag([1;-1;1])),...\n              mirrorh(diag([1;-1;1])),...\n              mirrorh(diag([1;-1;1])),...\n              diag([-1;-1;1]),...\n              diag([-1;-1;1]),...\n              diag([-1;-1;1]),...\n              diag([-1;-1;1]),...\n              mirrorh(diag([-1;-1;-1])),...\n              mirrorh(diag([-1;-1;-1])),...\n              mirrorh(diag([-1;-1;-1])),...\n              mirrorh(diag([-1;-1;-1])),... \n              diag([1;-1;-1]),...\n              diag([1;-1;-1]),...\n              diag([1;-1;-1]),...\n              diag([1;-1;-1])];\npm_init = [0;0;0;pi/2;-pi/2;0.04];\nB_earth = [-0.553111111\t-0.374555556\t-0.122619048...\n-0.515809524\t-0.295809524\t-0.077047619...\n-0.636904762\t-0.354634921\t-0.125174603...\n-0.544126984\t-0.318142857\t-0.118666667...\n0.235396825\t-0.012873016\t-0.451079365...\n0.087587302\t-0.320460317\t-0.478063492...\n0.075079365\t-0.297063492\t-0.457571429...\n0.078126984\t-0.341047619\t-0.499793651...\n0.401380952\t-0.248206349\t0.061952381...\n0.469435484\t-0.180274194\t0.06766129...\n0.442419355\t-0.269870968\t0.077758065...\n0.489177419\t-0.270806452\t-0.108483871...\n0.009730159\t-0.086761905\t0.67131746...\n-0.059096774\t-0.115145161\t0.576403226...\n-0.076854839\t-0.088258065\t0.584709677...\n-0.100354839\t-0.071241935\t0.519322581]';\nB_earth = [-0.567333\t\t-0.364333\t\t-0.155...\n-0.535667\t-0.278667\t\t-0.131...\n-0.669\t\t-0.355333\t\t-0.165...\n-0.562\t\t-0.300667\t\t-0.163667...\n0.278333\t-0.006\t\t-0.464333...\n0.126667\t-0.311\t\t-0.51...\n0.117667\t-0.29\t\t-0.499333...\n0.116\t\t-0.326667\t\t-0.534333...\n0.468667\t-0.243667\t\t0.04...\n0.506667\t-0.171667\t\t0.116...\n0.476\t\t-0.279333\t\t0.0543333...\n0.538667\t-0.255\t\t-0.0236667...\n-0.0566667\t-0.0843333\t\t0.678667...\n-0.126667\t-0.107667\t\t0.598333...\n-0.147333\t-0.0766667\t\t0.605...\n-0.172333\t-0.0466667\t\t0.542]';"() -> ("meas_dir_s"=w38:i32[][], "xyz_s"=w37:dbl[][], "pm_init"=w33:dbl[], "B_earth"=w32:dbl[])  [unwired: 1 in, 1 out]
      n29 = case shown="True" "Bifur?" {
        tunnel: [w41 w180] -> w27
        frame False {
          n30 = mathscript code="% line 1\ny1=[-35:0.1:0];\nx1=sqrt(35.92^2-(y1+17.5).^2)-26.37-1;\n\ny2=[-35:0.1:0];\nx2 =sqrt(35.92^2-(y1+17.5).^2)-26.37-10+1;\n\ny3 = [0:0.1:35];\nx3 = -sqrt(35.92^2-(y3-17.5).^2)+36.37-1;\n\ny4 = [0:0.1:35];\nx4 = -sqrt(35.92^2-(y4-17.5).^2)+36.37-10+1;"() -> ("y1"=w53:dbl[], "x1"=w52:cdb[], "y2"=w50:dbl[], "x2"=w49:cdb[], "y3"=w48:dbl[], "x3"=w47:cdb[], "y4"=w46:dbl[], "x4"=w45:cdb[])  [unwired: 1 in, 1 out]
          n31 = Bundle("y1"=w53, "x1"=w52) -> (w51:cluster{"y1":dbl[], "x1":cdb[]})  [unwired: 1 in]
          n32 = Bundle("y2"=w50, "x2"=w49) -> (w44:cluster{"y2":dbl[], "x2":cdb[]})  [unwired: 1 in]
          n33 = Bundle("y3"=w48, "x3"=w47) -> (w43:cluster{"y3":dbl[], "x3":cdb[]})  [unwired: 1 in]
          n34 = Bundle("y4"=w46, "x4"=w45) -> (w42:cluster{"y4":dbl[], "x4":cdb[]})  [unwired: 1 in]
          n35 = Build Array(w51, w44, w43, w42) -> (w41:cluster{"y4":dbl[], "x4":cdb[]}[])
        }
        frame True {
          # "For plotting"
          n36 = mathscript code="width = 8;\nW = 32;\nlen = 88;\noffset=-10;\n% line 1\ny1_1 = [1.5:0.1:89.5];\ny1 = y1_1-offset;\nx1 = -width/2*ones(1,length(y1_1));\nk11 = 25/(W-width)*2;\ny11_1 = [(1.5):-0.1:(1.5-25)];\ny11 = y11_1 - offset;\nx11 = -width/2-((89.5-len)-y11_1)/k11;\n\n% line 2\ny2_1 = [1.5:0.1:89.5];\ny2 = y2_1 - offset;\nx2 = width/2*ones(1,length(y2_1));\nk22 = 28/(W-width)*2;\ny22_1 = [1.5:-0.1:(1.5-28)];\ny22 = y22_1-offset;\nx22 = width/2+((89.5-len)-y11_1)/k11;\n\n% line 3\ny3_1 = [(1.6-16):-0.1:(1.6-16-33.333)];\ny3 = y3_1-offset;\nx3 = -(1.6-16-y3_1)/k11;\n\n% line 4\ny4_1 = [(1.6-16):-0.1:(1.6-16-33.333)];\ny4 = y4_1-offset;\nx4 = (1.6-16-y4_1)/k11;"() -> ("y1"=w198:dbl[], "x1"=w197:dbl[], "y11"=w196:dbl[], "x11"=w195:dbl[], "y2"=w192:dbl[], "x2"=w191:dbl[], "y22"=w189:dbl[], "x22"=w188:dbl[], "y3"=w186:dbl[], "x3"=w185:dbl[], "y4"=w183:dbl[], "x4"=w182:dbl[])  [unwired: 1 in, 1 out]
          n37 = Bundle("y1"=w198, "x1"=w197) -> (w194:cluster{"y1":dbl[], "x1":dbl[]})  [unwired: 1 in]
          n38 = Bundle("y11"=w196, "x11"=w195) -> (w193:cluster{"y11":dbl[], "x11":dbl[]})  [unwired: 1 in]
          n39 = Bundle("y2"=w192, "x2"=w191) -> (w190:cluster{"y2":dbl[], "x2":dbl[]})  [unwired: 1 in]
          n40 = Bundle("y22"=w189, "x22"=w188) -> (w187:cluster{"y22":dbl[], "x22":dbl[]})  [unwired: 1 in]
          n41 = Bundle("y3"=w186, "x3"=w185) -> (w184:cluster{"y3":dbl[], "x3":dbl[]})  [unwired: 1 in]
          n42 = Bundle("y4"=w183, "x4"=w182) -> (w181:cluster{"y4":dbl[], "x4":dbl[]})  [unwired: 1 in]
          n43 = Build Array(w194, w193, w190, w187, w184, w181) -> (w180:cluster{"y4":dbl[], "x4":dbl[]}[])
        }
      }
      n44 = Initialize Array(0.0 ("element"), 0 ("dimension size")) -> (w26:dbl[])
      n45 = Initialize Array(0.0 ("element"), 0 ("dimension size")) -> (w25:dbl[])
      n46 = Initialize Array(0.0 ("element"), 48 ("dimension size")) -> (w34:dbl[])
    }
    frame #1 {
      # "Plotting"
      n47 = while {
        shift-right: [w3324] -> _
        shift-left: w991 -> [w3319]
        shift-right: [w3325] -> _
        shift-left: w992 -> [w3316]
        tunnel: w993 -> [w3321]
        tunnel: w991 -> [w3314]
        stop <- w3320 stop-if-true
        n48 = local read "Action Mode"() -> (w3322:T1)
        n49 = call "Wait"("Count(mSec)"=u32 250) -> ()  [unwired: 1 out]
        n50 = Select(t=w3314, s="Clear plot?", f=w3319) -> (s? t:f=w3318:dbl[])
        n51 = Select(t=w3314, s="Clear plot?", f=w3316) -> (s? t:f=w3315:dbl[])
        n52 = case shown="\"Sensing\", Default" w3322 {
          tunnel: w3318 -> [w3401 w3406 w3424]
          tunnel: w3315 -> [w3402 w3407 w3423]
          tunnel: [w3402 w3407 w3422] -> w3325
          tunnel: [w3401 w3406 w3421] -> w3324
          tunnel: [w3404 w3409 w3416] -> w3323
          tunnel: w3321 -> [w3403 w3408 w3411]
          frame "Actuation" {
            n53 = Bundle(w3402, w3401) -> (w3405:cluster{dbl[], dbl[]})  [unwired: 1 in]
            n54 = Build Array (concatenate)(w3405, w3403) -> (w3404:cluster{"y4":dbl[], "x4":cdb[]}[])
          }
          frame "Waiting" {
            n55 = Bundle(w3407, w3406) -> (w3410:cluster{dbl[], dbl[]})  [unwired: 1 in]
            n56 = Build Array (concatenate)(w3410, w3408) -> (w3409:cluster{"y4":dbl[], "x4":cdb[]}[])
          }
          frame "Sensing", Default {
            # "X"
            # "Y"
            n57 = local read "pm_hat_opt"() -> (w3414:dbl[])
            n58 = Index Array(array=w3414, index #1=0 ("index"), index #2=1 ("index")) -> (element #1=w3413:dbl, element #2=w3412:dbl)
            n59 = Multiply(x=1000.0, y=w3413) -> (x*y=w3417:dbl)
            n60 = Multiply(x=w3412, y=-1000.0) -> (x*y=w3419:dbl)
            n61 = Build Array (concatenate)(w3424, w3417) -> (w3421:dbl[])
            n62 = Build Array (concatenate)(w3423, w3419) -> (w3422:dbl[])
            n63 = Bundle(w3422, w3421) -> (w3415:cluster{dbl[], dbl[]})  [unwired: 1 in]
            n64 = Build Array (concatenate)(w3415, w3411) -> (w3416:cluster{"y4":dbl[], "x4":cdb[]}[])
          }
        }
        "XY Graph" <- w3323
        n65 = xnode "Stepper position"() -> ("C/AI0 (AI0)"=→"Encoder 1 AI0":dbl)  [unwired: 1 in, 1 out]
        n66 = xnode "Analog input (1 sample)"() -> ("C/AI1 (AI1)"=→"Encoder 2 AI1":dbl)  [unwired: 1 in, 1 out]
        n67 = local read "stop"() -> (w3320:bool)
      }
      n68 = local read "Update M in realtime?"() -> (w988:bool)
      n69 = case shown="False" w988 {
        tunnel: [w998 w1010] -> w989
        tunnel: w990 -> [w1009 w1010]
        frame False {
          n70 = Index Array(array=w1009, index #1=0 ("index"), index #2=1 ("index"), index #3=2 ("index"), index #4=3 ("index"), index #5=4 ("index")) -> (element #1=w1003:dbl, element #2=w1002:dbl, element #3=w1001:dbl, element #4=w1000:dbl, element #5=w999:dbl)
          n71 = Build Array(w1003, w1002, w1001, w1000, w999) -> (w998:dbl[])
        }
        frame True {
        }
      }
      n72 = while {
        shift-right: [w1013] -> _
        shift-left: w997 -> [w1019]
        shift-right: [w1018] -> _
        shift-left: w989 -> [w1017]
        tunnel: w996 -> [w1016]
        tunnel: w995 -> [w1015]
        tunnel: w994 -> [w1014]
        stop <- "stop" stop-if-true
        n73 = case shown="\"Actuation\"" "Action Mode" {
          tunnel: w1019 -> [w1021 w1099 w1148]
          tunnel: [w1020 w1100 w1147] -> w1018
          tunnel: w1017 -> [w1020 w1100 w1146]
          tunnel: w1016 -> [_ _ w1145]
          tunnel: w1015 -> [_ _ w1144]
          tunnel: w1014 -> [_ _ w1143]
          tunnel: [w1021 w1099 w1142] -> w1013
          frame "Actuation" {
            n74 = flat-sequence {
              frame #0 {
                n75 = call "Wait2"("Count(uSec)"=u32 1000 ("Count(mSec)")) -> ()  [unwired: 1 out]
                n76 = Select(t="Actuation Current", s="Actuation on?", f=0.0) -> (s? t:f=w1024:dbl)
                n77 = Absolute Value(x=w1024) -> (abs(x)=w1025:dbl)
                n78 = Greater Than 0?(x=w1024) -> (x > 0?=w1023:bool)
                n79 = xnode "PWM 2"("Duty Cycle"=w1025) -> ()  [unwired: 1 in, 1 out]
                n80 = xnode "Digital output (1 sample)"("C/DIO2 (DIO2)"=w1023) -> ()  [unwired: 1 in, 1 out]
              }
            }
          }
          frame "Waiting" {
            # "Change to next Sensing mode"
            # "Gradually decrease to zero"
            # "wait for field to disappear"
            n81 = flat-sequence {
              frame #0 {
                n82 = local write "Actuation on?"(FALSE ("Actuation on?")) -> ()
                n83 = call "Wait3"("Count(mSec)"=u32 60) -> ()  [unwired: 1 out]
                n84 = local read "Actuation Current"() -> (w1101:dbl)
                n85 = xnode "PWM"("Duty Cycle"=w1101) -> ()  [unwired: 1 in, 1 out]
              }
            }
          }
          frame "Sensing", Default {
            n86 = call "Tick Count"() -> ("Tick Count(uSec)"=w1141:u32)
            n87 = flat-sequence {
              tunnel: [w1151] -> w1149
              tunnel: w1148 -> [w1150]
              tunnel: w1149 -> [w1390]
              tunnel: [w1395] -> w1147
              tunnel: w1146 -> [w1394]
              tunnel: w1145 -> [w1393]
              tunnel: w1144 -> [w1392]
              tunnel: w1143 -> [w1391]
              tunnel: [w1390] -> w1142
              frame #0 {
                # "Run 8 Iterations to read all sensors data simultaneously"
                n88 = for {
                  N: 8 -> [_]
                  shift-right: [w1164] -> w1151
                  shift-left: w1150 -> [w1166]
                  i -> [w1167]
                  # "B_meas"
                  n89 = Decrement(x=w1167) -> (x-1=w1160:i32)
                  n90 = Quotient & Remainder(x=w1160, y=8) -> (x-y*floor(x/y)=w1168:i32)  [unwired: 1 out]
                  n91 = Less Or Equal?(x=w1160, y=3) -> (x <= y?=w1158:bool)
                  n92 = Multiply(x=w1160, y=3) -> (x*y=w1157:i32)
                  n93 = Scale By Power Of 2(n=w1168, x=1) -> (x*2^n=w1169:i32)
                  n94 = Select(t=0, s=w1158, f=24) -> (s? t:f=w1154:i32)
                  n95 = Add(x=w1157, y=12) -> (x+y=w1161:i32)
                  n96 = Add(x=w1157, y=w1154) -> (x+y=w1153:i32)
                  n97 = Build Array(w1169) -> (w1171:i32[])
                  n98 = flat-sequence {
                    tunnel: w1171 -> [w1184]
                    tunnel: [w1184] -> w1174
                    tunnel: [w1182] -> w1173
                    tunnel: w1166 -> [w1178]
                    tunnel: [w1177] -> w1165
                    tunnel: w1161 -> [w1175]
                    tunnel: w1174 -> [w1291]
                    tunnel: w1173 -> [w1289]
                    tunnel: w1165 -> [w1288]
                    tunnel: [w1287] -> w1164
                    tunnel: w1153 -> [w1282]
                    frame #0 {
                      w1193 = i16 3000  # Gain Lsb/G
                      # "Sensor 5,6,7,8,9,10,11,12"
                      # "Z"
                      # "Y"
                      # "X"
                      n99 = xnode "I2C Multiplex 2"("Slave Address (7-bit)"=u8 112, "Bytes to Write"=w1184) -> ("error out"=w1183:errorcluster)  [unwired: 1 in]
                      n100 = Build Array(u8 0) -> (w1197:u8[])
                      n101 = xnode "I2C 2"("Slave Address (7-bit)"=u8 13, "Bytes to Write"=w1197, "Byte Count"=u32 6, "error in (no error)"=w1183) -> ("Bytes Read"=w1200:u8[], "error out"=w1182:errorcluster)
                      n102 = Index Array(array=w1200) -> (element #1=w1192:u8, element #2=w1191:u8, element #3=w1189:u8, element #4=w1190:u8, element #5=w1187:u8, element #6=w1188:u8)  [unwired: 6 in]
                      n103 = Join Numbers(hi=w1191, lo=w1192) -> ((hi.lo)=w1203:u16)
                      n104 = Join Numbers(hi=w1190, lo=w1189) -> ((hi.lo)=w1201:u16)
                      n105 = Join Numbers(hi=w1188, lo=w1187) -> ((hi.lo)=w1202:u16)
                      n106 = To Word Integer(number=w1203) -> (16bit integer=w1196:i16)
                      n107 = To Word Integer(number=w1201) -> (16bit integer=w1195:i16)
                      n108 = To Word Integer(number=w1202) -> (16bit integer=w1194:i16)
                      n109 = Divide(x=w1196, y=w1193) -> (x/y=w1181:dbl)
                      n110 = Divide(x=w1195, y=w1193) -> (x/y=w1180:dbl)
                      n111 = Divide(x=w1194, y=w1193) -> (x/y=w1179:dbl)
                      n112 = Build Array(w1181, w1180, w1179) -> (w1176:dbl[])
                      n113 = Replace Array Subset(array=w1178, new element=w1176, index=w1175) -> (w1177:dbl[])
                    }
                    frame #1 {
                      w1300 = i16 3000  # Gain Lsb/G
                      # "Sensor 1,2,3,4,13,14,15,16"
                      n114 = xnode "I2C Multiplex 3"("Slave Address (7-bit)"=u8 113, "Bytes to Write"=w1291, "error in (no error)"=w1289) -> ("error out"=w1290:errorcluster)
                      n115 = Build Array(u8 0) -> (w1304:u8[])
                      n116 = xnode "I2C"("Slave Address (7-bit)"=u8 13, "Bytes to Write"=w1304, "Byte Count"=u32 6, "error in (no error)"=w1290) -> ("Bytes Read"=w1307:u8[])  [unwired: 1 out]
                      n117 = Index Array(array=w1307) -> (element #1=w1299:u8, element #2=w1298:u8, element #3=w1296:u8, element #4=w1297:u8, element #5=w1294:u8, element #6=w1295:u8)  [unwired: 6 in]
                      n118 = Join Numbers(hi=w1298, lo=w1299) -> ((hi.lo)=w1310:u16)
                      n119 = Join Numbers(hi=w1297, lo=w1296) -> ((hi.lo)=w1308:u16)
                      n120 = Join Numbers(hi=w1295, lo=w1294) -> ((hi.lo)=w1309:u16)
                      n121 = To Word Integer(number=w1310) -> (16bit integer=w1303:i16)
                      n122 = To Word Integer(number=w1308) -> (16bit integer=w1302:i16)
                      n123 = To Word Integer(number=w1309) -> (16bit integer=w1301:i16)
                      n124 = Divide(x=w1303, y=w1300) -> (x/y=w1286:dbl)
                      n125 = Divide(x=w1302, y=w1300) -> (x/y=w1285:dbl)
                      n126 = Divide(x=w1301, y=w1300) -> (x/y=w1284:dbl)
                      n127 = Build Array(w1286, w1285, w1284) -> (w1283:dbl[])
                      n128 = Replace Array Subset(array=w1288, new element=w1283, index=w1282) -> (w1287:dbl[])
                    }
                  }
                }
              }
              frame #1 {
                # "B_earth_field"
                n129 = Subtract(x=w1390, y=w1391) -> (x-y=w1396:dbl[])
                n130 = case shown="False" "Update M in realtime?" {
                  tunnel: w1396 -> [w1401 w2365]
                  tunnel: [w1397 w2364] -> w1395
                  tunnel: w1394 -> [w1398 w2363]
                  tunnel: w1393 -> [w1399 w2362]
                  tunnel: w1392 -> [w1400 w2361]
                  frame False {
                    n131 = mathscript code="pm_init = pm_init';\ny_meas = y_meas*1e-4;  % convert from Gauss to Tesla\nn_par = length(pm_init);\niteration = 0;  % current number of \nstop = 0;  % stop flag\nMaxIter = 100;   % maximum number of iteration\nepsilon_1 = 1e-10;  % convergence tolerance for gradient\nepsilon_2 = 1e-9;  % convergence tolerance for parameter\nepsilon_3 = 1e-15;  % convergence tolerance for residual error\nepsilon_4 = 1e-8;  % determines acceptance of a L-M step\npm = pm_init; % initialization on parameters\nlambda_0 = 1e-3;  % user-specified initial lambda\n% Jacobian initialization\nJ = Analytic_Jacobian_Mag_cir_array_noM(pm_init,xyz_s,meas_dir_s,M);\n% initialize L-M parameters\nlambda = lambda_0*max(diag(J'*J));\nv = 2;  % scale factor\nwhile ( ~stop)\n    iteration = iteration + 1;\n    B_meas = PM_forward_field_noM(pm,xyz_s,meas_dir_s,M);\n% compute residual error between model and measurement\n    err = (y_meas - B_meas)';\n    if ( norm(err)^2< epsilon_3 &&  iteration > 2 )\n        stop = 1;\n        break;\n    end\n    % compute gradient\n    grad = J'*err;\n    % check stopping criterion 1\n    if ( max(abs(grad)) < epsilon_1  &&  iteration > 2 )\n        stop = 1;\n        break\n    end\n    % parameter increment change\n    delta = (J'*J + lambda*eye(n_par))\\J'*err;  % simplest version\n    % check stopping criterion 2 \n    if ( max(abs(delta)./(abs(pm)+1e-20)) < epsilon_2  &&  iteration > 2 )\n        stop = 1;\n        break\n    end\n    pm_try = pm + delta;\n    % evaluate value using pm_try\n    B_meas_try = PM_forward_field_noM(pm_try,xyz_s,meas_dir_s,M);  % compute measurement based on given direction\n    err_try = (y_meas - B_meas_try)';\n    % compute rho for determining acceptance\n    rho = (err'*err - err_try'*err_try)/(delta'*(lambda*delta + J'*err) );\n    if rho > epsilon_4   % if better\n        pm = pm_try;  % accpet pm_try\n        lambda = lambda*max( 1/3, 1-(2*rho-1)^3 );\n        v = 2;\n             % update Jacobian matrix\n        J = Analytic_Jacobian_Mag_cir_array_noM(pm,xyz_s,meas_dir_s,M);\n    else      % if not better\n        lambda = lambda*v;\n        v = 2*v;\n    end\n    if ( iteration == MaxIter )\n        stop = 1;\n    end\nend\n\npm_hat_opt = pm;"("meas_dir_s"=w1400, "xyz_s"=w1399, "y_meas"=w1401, "pm_init"=w1398, "M"="M") -> ("pm_hat_opt"=w1397:dbl[])  [unwired: 1 in, 1 out]
                  }
                  frame True {
                    # "Use current optimal point as initial guess for next iteration"
                    n132 = mathscript code="pm_init = pm_init';\ny_meas = y_meas*1e-4;  % convert from Gauss to Tesla\nn_par = length(pm_init);\niteration = 0;  % current number of \nstop = 0;  % stop flag\nMaxIter = 100;   % maximum number of iteration\nepsilon_1 = 1e-10;  % convergence tolerance for gradient\nepsilon_2 = 1e-9;  % convergence tolerance for parameter\nepsilon_3 = 1e-15;  % convergence tolerance for residual error\nepsilon_4 = 1e-8;  % determines acceptance of a L-M step\npm = pm_init; % initialization on parameters\nlambda_0 = 1e-3;  % user-specified initial lambda\n% Jacobian initialization\nJ = Analytic_Jacobian_Mag_cir_array_test(pm_init,xyz_s,meas_dir_s);\n% initialize L-M parameters\nlambda = lambda_0*max(diag(J'*J));\nv = 2;  % scale factor\nwhile ( ~stop)\n    iteration = iteration + 1;\n    B_meas = PM_forward_field(pm,xyz_s,meas_dir_s);\n% compute residual error between model and measurement\n    err = (y_meas - B_meas)';\n    if ( norm(err)^2< epsilon_3 &&  iteration > 2 )\n        stop = 1;\n        break;\n    end\n    % compute gradient\n    grad = J'*err;\n    % check stopping criterion 1\n    if ( max(abs(grad)) < epsilon_1  &&  iteration > 2 )\n        stop = 1;\n        break\n    end\n    % parameter increment change\n    delta = (J'*J + lambda*eye(n_par))\\J'*err;  % simplest version\n    % check stopping criterion 2 \n    if ( max(abs(delta)./(abs(pm)+1e-20)) < epsilon_2  &&  iteration > 2 )\n        stop = 1;\n        break\n    end\n    pm_try = pm + delta;\n    % evaluate value using pm_try\n    B_meas_try = PM_forward_field(pm_try,xyz_s,meas_dir_s);  % compute measurement based on given direction\n    err_try = (y_meas - B_meas_try)';\n    % compute rho for determining acceptance\n    rho = (err'*err - err_try'*err_try)/(delta'*(lambda*delta + J'*err) );\n    if rho > epsilon_4   % if better\n        pm = pm_try;  % accpet pm_try\n        lambda = lambda*max( 1/3, 1-(2*rho-1)^3 );\n        v = 2;\n             % update Jacobian matrix\n        J = Analytic_Jacobian_Mag_cir_array_test(pm,xyz_s,meas_dir_s);\n    else      % if not better\n        lambda = lambda*v;\n        v = 2*v;\n    end\n    if ( iteration == MaxIter )\n        stop = 1;\n    end\nend\n\npm_hat_opt = pm;"("meas_dir_s"=w2361, "xyz_s"=w2362, "y_meas"=w2365, "pm_init"=w2363) -> ("pm_hat_opt"=w2364:dbl[])  [unwired: 1 in, 1 out]
                  }
                }
                "pm_hat_opt" <- w1395
              }
            }
            n133 = feedback #1() -> (w1140:u32)  [unwired: 1 in]
            n134 = feedback-in #1(w1141) -> ()
            n135 = Subtract(x=w1141, y=w1140) -> (x-y=→"Sensing time":u32)
          }
        }
      }
    }
    frame #2 {
      n136 = xnode "PWM 3"("Duty Cycle"=0.0) -> ()  [unwired: 1 in, 1 out]
    }
  }
